vi "Change Local Slots.vi"(8 "error in":errorcluster, 10 "# Slots":i32, 11 "Item Ref in":T1 format="%.0x") -> (0 "error out":errorcluster, 3 "Item Ref out":T1 format="%.0x")   [LabVIEW 2011, in "Scan Engine Custom Device.lvlib"]
uses:
  Scan Engine Custom Device.lvlib
  <vilib>/NI Veristand/Custom Device API/Custom Device Item Ref.ctl
  Modules.lvlibp/RSI Module/Module Models.ctl
  Modules.lvlibp/RSI Module/Slot Settings.ctl
  Globals/Property Strings.vi
  <vilib>/NI Veristand/Custom Device API/Get Item Property (I32).vi
  <vilib>/NI Veristand/Custom Device API/Set Item Property (I32).vi
  Globals/Scan Engine GUIDs.vi
  Modules.lvlibp/RSI Module/Class Property Strings.vi
  <vilib>/NI Veristand/Custom Device API/Custom Device API.lvlib
  Modules.lvlibp/RSI Module/RSI Module.lvclass
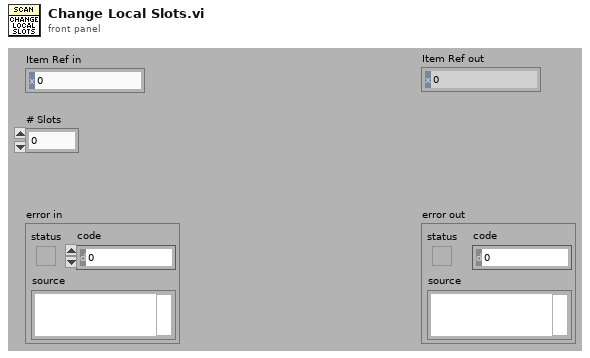
[diagram p1: front panel]
types:
  T1 = typedef "Custom Device API.lvlib/Custom Device Item Ref.ctl" = u64
  T2 = typedef "Modules.lvlibp/RSI Module.lvclass/Module Models.ctl" = enum16{"Empty", "NI 9201", "NI 9203", "NI 9205", "NI 9206", "NI 9207", "NI 9208", "NI 9211", "NI 9213", "NI 9214", "NI 9215", "NI 9217", "NI 9219", "NI 9221", "NI 9225", "NI 9227", "NI 9229", "NI 9233", "NI 9234", "NI 9235", "NI 9236", "NI 9237", "NI 9239", "NI 9263", "NI 9264", "NI 9265", "NI 9269", "NI 9375", "NI 9401", "NI 9402", "NI 9403", "NI 9411", "NI 9421", "NI 9422", "NI 9423", "NI 9425", "NI 9426", "NI 9435", "NI 9472", "NI 9474", "NI 9475", "NI 9476", "NI 9477", "NI 9478", "NI 9481", "NI 9482", "NI 9485"}
  T3 = typedef "Modules.lvlibp/RSI Module.lvclass/Slot Settings.ctl" = cluster{"Slot":u32, "EtherCAT?":bool}
  T4 = typedef "Custom Device API.lvlib/Custom Device Item Info.ctl" = cluster{"Name":string, "Is Channel":bool, "GUID":string}
  T5 = typedef "Modules.lvlibp/Custom Device API.lvlib/Custom Device Item Ref.ctl" = u64
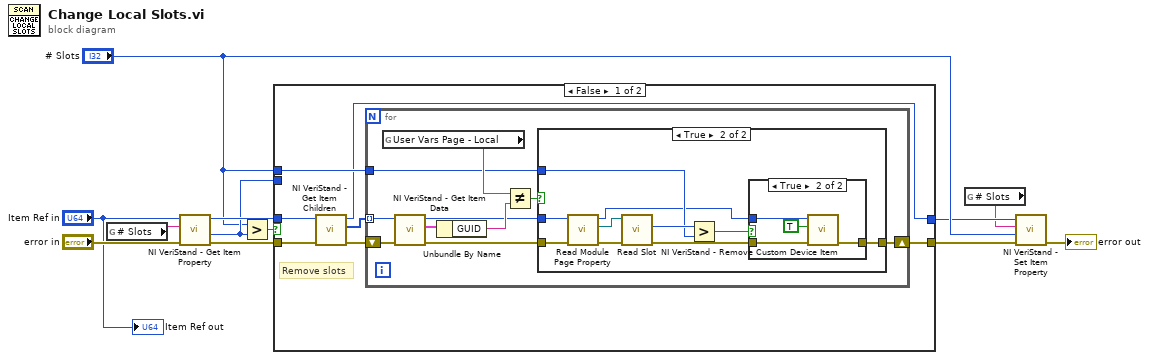
[diagram p0: block diagram]
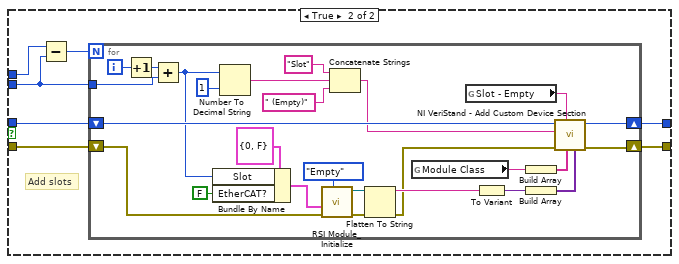
[diagram p4: hidden frame]
diagram:
  n1 = global read "Property Strings.vi" "# Slots"() -> (w8:string)
  n2 = call-poly <vilib>:"NI VeriStand - Get Item Property.vi"("error in (no error)"="error in", "Property Name"=w8, "Item Ref in"="Item Ref in") -> ("error out"=w12:errorcluster, "Value"=w6:i32, "Item Ref out"=w11:T1)  [unwired: 5 in, 1 out]
  n3 = Greater?(x="# Slots", y=w6) -> (0:w10:bool)
  n4 = case shown="False" w10 {
    tunnel: w11 -> [w19 w48]
    tunnel: w12 -> [w18 w51]
    tunnel: [w15 w47] -> w5
    tunnel: "# Slots" -> [w14 w52]
    tunnel: w6 -> [_ w49]
    tunnel: [w13 w46] -> w2
    frame False {
      # "Remove slots"
      n5 = call <vilib>:"NI VeriStand - Get Item Children.vi"("error in (no error)"=w18, "Item Ref in"=w19) -> ("error out"=w16:errorcluster, "Child Refs"=w17:T1[], "Item Ref out"=w13:T1)  [unwired: 6 in, 1 out]
      n6 = for {
        tunnel: w17 -> [w28] mode=indexing
        shift-right: [w20] -> w15
        shift-left: w16 -> [w29]
        tunnel: w14 -> [w21]
        n7 = global read "Scan Engine GUIDs.vi" "User Vars Page - Local"() -> (w25:string)
        n8 = call <vilib>:"NI VeriStand - Get Item Data.vi"("error in (no error)"=w29, "Item Ref in"=w28) -> ("error out"=w22:errorcluster, "Item Info"=w27:T4, "Item Ref out"=w23:T1)  [unwired: 6 in, 1 out]
        n9 = Unbundle By Name(w27) -> ("GUID"=w26:string)
        n10 = Not Equal?(x=w25, y=w26) -> (x != y?=w24:bool)
        n11 = case shown="True" w24 {
          tunnel: w23 -> [_ w39]
          tunnel: w22 -> [w30 w40]
          tunnel: w21 -> [_ w35]
          tunnel: [w30 w31] -> w20
          frame False {
          }
          frame True {
            n12 = call "Read Module Page Property.vi"("error in (no error)"=w40, "Node Ptr In"=w39) -> ("error out"=w38:errorcluster, "RSI Module"=w37:refnum<class "RSI Module.lvclass">, "Node Ptr Out"=w32:T5)  [unwired: 7 in]
            n13 = call "Read Slot.vi"("error in (no error)"=w38, "RSI Module in"=w37) -> ("error out"=w33:errorcluster, "Slot"=w36:u32)  [unwired: 7 in, 1 out]
            n14 = Greater?(x=w36, y=w35) -> (0:w34:bool)
            n15 = case shown="True" w34 {
              tunnel: w33 -> [w41 w45]
              tunnel: w32 -> [_ w44]
              tunnel: [w41 w42] -> w31
              frame False {
              }
              frame True {
                n16 = call <vilib>:"NI VeriStand - Remove Custom Device Item.vi"("error in (no error)"=w45, "Force Delete (F)"=TRUE, "Item Ref in"=w44) -> ("error out"=w42:errorcluster)  [unwired: 7 in, 1 out]
              }
            }
          }
        }
      }
    }
    frame True {
      # "Add slots"
      n17 = Subtract(x=w52, y=w49) -> (x-y=w50:i32)
      n18 = for {
        N: w50 -> [_]
        shift-right: [w73] -> w47
        shift-left: w51 -> [w66]
        shift-right: [w72] -> w46
        shift-left: w48 -> [w78]
        tunnel: w49 -> [w54]
        i -> [w75]
        n19 = Increment(x=w75) -> (x+1=w55:i32)
        n20 = Add(x=w55, y=w54) -> (x+y=w53:i32)
        n21 = Bundle By Name(cluster=T3 {"Slot"=0, "EtherCAT?"=FALSE} ("Slot Settings"), "Slot"=w53, "EtherCAT?"=FALSE) -> (w69:T3)
        n22 = Number To Decimal String(number=w53, width (-)=i16 1) -> (decimal integer string=w77:string)
        n23 = call "RSI Module_Initialize.vi"("Module Model"=Module_Models."Empty" ("Module"), "error in (no error)"=w66, "Slot Settings"=w69) -> ("error out"=w59:errorcluster, "RSI Module out"=w61:refnum<class "RSI Module.lvclass">)  [unwired: 7 in]
        n24 = Concatenate Strings("Slot" ("string"), w77, " (Empty)" ("Section Name")) -> (w74:string)
        n25 = Flatten To String(anything=w61, error in (no error)=w59) -> (data string=w60:string, error out=w58:errorcluster)  [unwired: 2 in, 1 out]
        n26 = global read "Class Property Strings.vi" "Module Class"() -> (w57:string)
        n27 = global read "Scan Engine GUIDs.vi" "Slot - Empty"() -> (w62:string)
        n28 = To Variant(anything=w60) -> (Variant=w70:variant)
        n29 = Build Array(w57) -> (w65:string[])
        n30 = Build Array(w70) -> (w71:variant[])
        n31 = call <vilib>:"NI VeriStand - Add Custom Device Section.vi"("Property Values"=w71, "Property names"=w65, "GUID (Default Section)"=w62, "error in (no error)"=w58, "Section Name"=w74, "Parent Ref in"=w78) -> ("error out"=w73:errorcluster, "Parent Ref out"=w72:T1)  [unwired: 2 in, 2 out]
      }
    }
  }
  n32 = global read "Property Strings.vi" "# Slots"() -> (w1:string)
  n33 = call-poly <vilib>:"NI VeriStand - Set Item Property.vi"("error in (no error)"=w5, "Value"="# Slots", "Property Name"=w1, "Item Ref in"=w2) -> ("error out"=→"error out":errorcluster)  [unwired: 5 in, 2 out]
  "Item Ref out" <- "Item Ref in"
